vi "LED COM Reconnect.vi"(8 "error in (no error)":errorcluster, 11 "Queue in":refnum<queue>) -> (0 "error out":errorcluster)   [LabVIEW 2020]
uses:
  typedefs/LED Controller Messages.ctl
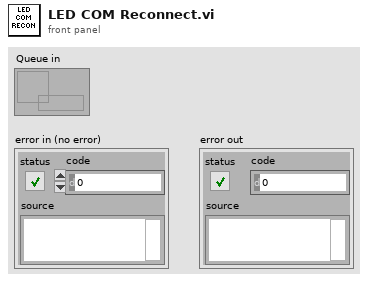
[diagram p1: front panel]
types:
  T1 = typedef "LED Controller Messages.ctl" = enum16{"Connect", "Disconnect", "Exit", "Set Mode A", "Set Mode B", "Set Range A", "Set Range B", "Set Output A", "Set Output B"}
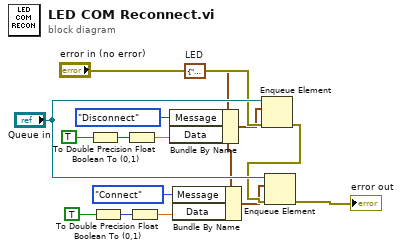
[diagram p0: block diagram]
diagram:
  w11 = cluster{"Message":T1, "Data":dbl} {"Message"=enum."Set Output B", "Data"=0.0}  # LED
  n1 = Boolean To (0,1)(Boolean=TRUE) -> (0, 1=w5:i16)
  n2 = Boolean To (0,1)(Boolean=TRUE) -> (0, 1=w6:i16)
  n3 = To Double Precision Float(number=w5) -> (double precision float=w4:dbl)
  n4 = To Double Precision Float(number=w6) -> (double precision float=w7:dbl)
  n5 = Bundle By Name(cluster=w11, "Message"=LED_Controller_Messages."Disconnect", "Data"=w4) -> (w3:cluster{"Message":T1, "Data":dbl})
  n6 = Bundle By Name(cluster=w11, "Message"=LED_Controller_Messages."Connect", "Data"=w7) -> (w8:cluster{"Message":T1, "Data":dbl})
  n7 = Enqueue Element(queue="Queue in", element=w3, error in (no error)="error in (no error)") -> (error out=w12:errorcluster)  [unwired: 1 in, 2 out]
  n8 = Enqueue Element(queue="Queue in", element=w8, error in (no error)=w12) -> (error out=→"error out":errorcluster)  [unwired: 1 in, 2 out]
